vi "logic_IO.vi"() -> ()   [LabVIEW 2018]
panel:
  out "decision":string
  in  "OK Button":bool
  in  "Cancel Button":bool
  out "Outcome":bool
  out "Boolean 2":bool=TRUE
  in  "Stop Button":bool=TRUE
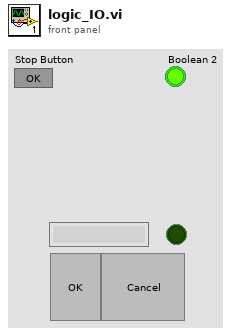
[diagram p1: front panel]
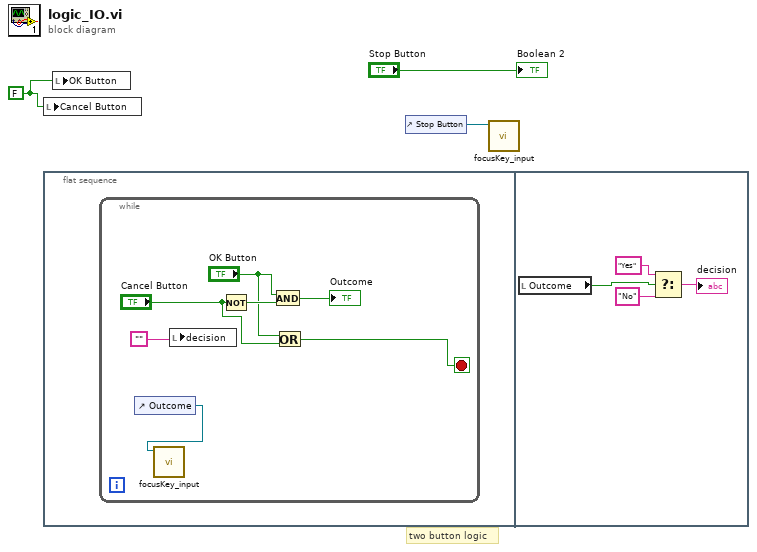
[diagram p0: block diagram]
diagram:
  w1 = FALSE
  # "two button logic"
  n1 = local write "Cancel Button"(w1) -> ()
  n2 = flat-sequence {
    frame #0 {
      n3 = while {
        stop <- w5 stop-if-true
        n4 = control-ref of="Outcome"() -> (w4:refnum<vi>)
        n5 = call "focusKey_input.vi"("reference"=w4) -> ()  [unwired: 10 in, 1 out]
        n6 = local write "decision"("") -> ()
        n7 = Not(x="Cancel Button") -> (.not. x?=w10:bool)
        n8 = And(x="OK Button", y=w10) -> (x .and. y?=→"Outcome":bool)
        n9 = Or(x="OK Button", y="Cancel Button") -> (x .or. y?=w5:bool)
      }
    }
    frame #1 {
      n10 = local read "Outcome"() -> (w14:bool)
      n11 = Select(t="Yes", s=w14, f="No") -> (s? t:f=→"decision":string)
    }
  }
  n12 = local write "OK Button"(w1) -> ()
  n13 = control-ref of="Stop Button"() -> (w3:refnum<vi>)
  n14 = call "focusKey_input.vi"("reference"=w3) -> ()  [unwired: 10 in, 1 out]
  "Boolean 2" <- "Stop Button"
